vi "Filter Inherited.vi"(8 "error in (no error)":errorcluster, 11 "LUnit Test Suite in":refnum<class "LUnit Test Suite.lvclass">) -> (0 "error out":errorcluster, 3 "LUnit Test Suite out":refnum<class "LUnit Test Suite.lvclass">)   [LabVIEW 2020, in "Execution UI.lvclass"]
uses:
  Execution UI.lvclass
  Execution UI.lvclass/Execution UI.ctl
  API/LUnit Test Suite/LUnit Test Suite.lvclass
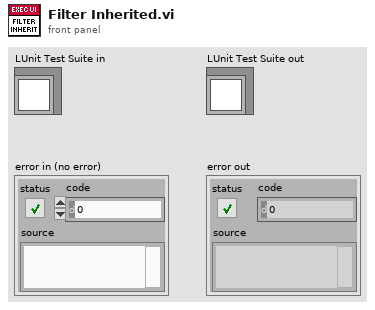
[diagram p1: front panel]
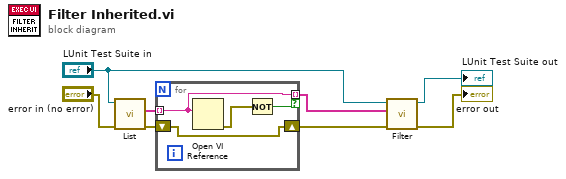
[diagram p0: block diagram]
diagram:
  n1 = call-dynamic "List.vi"("error in (no error)"="error in (no error)", "LUnit Test Suite In"="LUnit Test Suite in") -> ("error out"=w4:errorcluster, "List of Runnables"=w6:string[])  [unwired: 8 in]
  n2 = for {
    tunnel: w6 -> [w12] mode=indexing
    tunnel: [w12] -> w7 mode=indexing if=w10
    shift-right: [w9] -> w3
    shift-left: w4 -> [w9]
    n3 = Open VI Reference(vi path=w12) -> (error out=w11:errorcluster)  [unwired: 5 in, 1 out]
    n4 = Not(x=w11) -> (.not. x?=w10:bool)
  }
  n5 = call-dynamic "Filter.vi"("error in (no error)"=w3, "Selected Runnables"=w7, "LUnit Test Suite In"="LUnit Test Suite in") -> ("error out"=→"error out":errorcluster, "LUnit Test Suite Out"=→"LUnit Test Suite out":refnum<class "LUnit Test Suite.lvclass">)  [unwired: 7 in]
